vi "UV-VIS GetAcquiredData.vi"(4 "error in (no error)":errorcluster, 6 "size":u32, 7 "Detector in":refnum<class "UV-VIS.lvclass">) -> (0 "error out":errorcluster, 1 "DLL error code":u32, 2 "array":i32[](array[numeric]), 3 "Detector out":refnum<class "UV-VIS.lvclass">)   [LabVIEW 2015, in "UV-VIS.lvclass"]
doc: "This function will return the data from the last acquisition. The data are returned as long integers (32-bit signed integers).\n\n<B>Parameters</B>:\nsize - total number of pixels.\narray - data storage.\n\n<B>Error codes:</B>\nDRV_SUCCESS - Data copied.\nDRV_NOT_INITIALIZED - System not initialized.\nDRV_ACQUIRING - Acquisition in progress.\nDRV_ERROR_ACK - Unable to communicate with card.\nDRV_P1INVALID - Invalid pointer (i.e. NULL).\nDRV_P2INVALID - Array size is too small."
uses:
  UV-VIS.lvclass
  Detector.lvclass/Detector.ctl
  Detector.lvclass
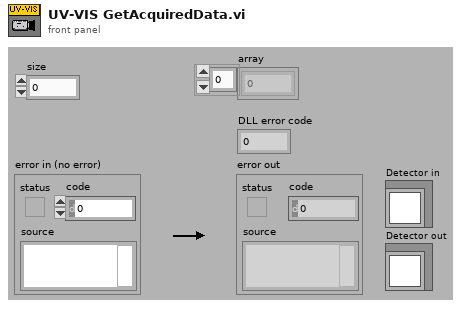
[diagram p1: front panel]
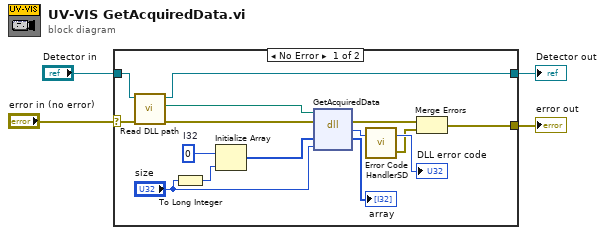
[diagram p0: block diagram]
diagram:
  n1 = case shown="No Error" "error in (no error)" {
    selector: "error in (no error)" -> [w16 w21]
    tunnel: [w19 w21] -> w3
    tunnel: [w5 w20] -> w2
    tunnel: "Detector in" -> [w15 w20]
    frame No Error {
      w7 = 0  # I32
      n2 = call "Read DLL path.vi"("error in (no error)"=w16, "Detector in"=w15) -> ("error out"=w17:errorcluster, "DLL path"=w18:path, "Detector out"=w5:refnum<class "UV-VIS.lvclass">)  [unwired: 7 in]
      n3 = To Long Integer(number="size") -> (32bit integer=w6:i32)
      n4 = Initialize Array "Initialize Array"(w7, w6) -> (w10:i32[])
      n5 = dll-call lib="PTH2.abs GSDTRANCONDLLatmcd32d°extra.dll" fn="GetAcquiredData"(path in=w18, error in=w17, "array"=w10, "size"="size") -> (error out=w8:errorcluster, "return type"=w14:u32, "array"=→"array":i32[])  [unwired: 2 in, 1 out]
      n6 = call "Error Code HandlerSD.vi"("DLL error code"=w14) -> ("error out"=w9:errorcluster, "dup DLL error code"=→"DLL error code":u32)  [unwired: 1 in]
      n7 = Merge Errors(w8, w9) -> (w19:errorcluster)
    }
    frame Error {
    }
  }
  "error out" <- w3
  "Detector out" <- w2
